vi "Serial Read Flush.vi"(11 "IO Cluster In":T1={"Error"={"status"=FALSE, "code"=0, "source"=""}, "Encoder Calibration Values"=[22, 216], "Update Calibration"=FALSE, "JPEG Resolutions"=3, "Raw Resolutions"=1, "Image Mode"=enum."RAW Gray Scale", "FPGA Ref"=refnum} {"JPEG Resolutions" items=["160x128"=3, "320x240"=5, "640x480"=7]; "Raw Resolutions" items=["80x60"=1, "160x120"=3, "128x128"=9, "128x96"=11]}) -> (3 "IO Cluster Out":T1={"Error"={"status"=FALSE, "code"=0, "source"=""}, "Encoder Calibration Values"=[22, 216], "Update Calibration"=FALSE, "JPEG Resolutions"=3, "Raw Resolutions"=1, "Image Mode"=enum."RAW Gray Scale", "FPGA Ref"=refnum} {"JPEG Resolutions" items=["160x128"=3, "320x240"=5, "640x480"=7]; "Raw Resolutions" items=["80x60"=1, "160x120"=3, "128x128"=9, "128x96"=11]})   [LabVIEW 2019]
uses:
  QNET MS IO Cluster.ctl
  <vilib>/Utility/error.llb/Error Cluster From Error Code.vi
  <vilib>/rvi/errors/niLvFpgaAdjustHostInterfaceError.vi
  <vilib>/rvi/interface/nirviMethod/nirviMethod.xnode
  <vilib>/FPGAPlugInAG/Dynamic/niLvFpga_ReadFifo_Dynamic.vi
  <vilib>/rvi/errors/niLvFpgaMergeErrorWithErrorCode.vi
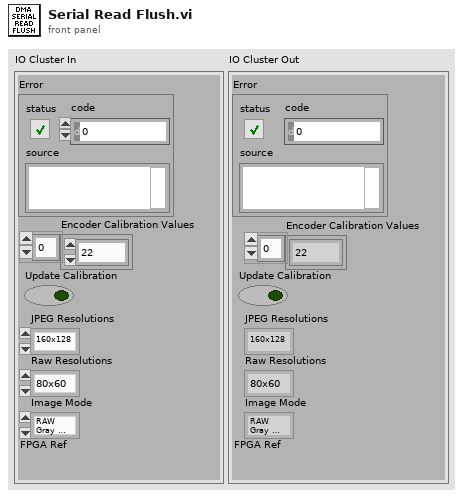
[diagram p1: front panel]
types:
  T1 = typedef "QNET MS IO Cluster.ctl" = cluster{"Error":errorcluster, "Encoder Calibration Values":i32[], "Update Calibration":bool, "JPEG Resolutions":u16, "Raw Resolutions":u16, "Image Mode":enum16{"RAW RGB", "RAW Gray Scale", "JPEG"}, "FPGA Ref":refnum<k20>}
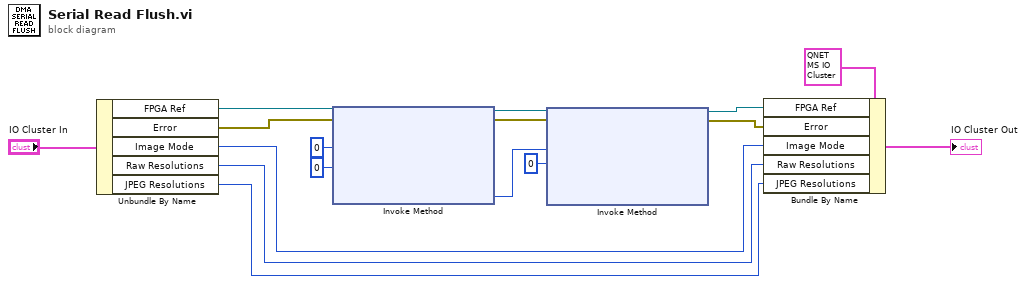
[diagram p0: block diagram]
diagram:
  n1 = Unbundle By Name("IO Cluster In") -> ("FPGA Ref"=w10:refnum<k20>, "Error"=w9:errorcluster, "Image Mode"=w6:enum16{"RAW RGB", "RAW Gray Scale", "JPEG"}, "Raw Resolutions"=w5:u16, "JPEG Resolutions"=w4:u16)
  n2 = xnode "Invoke Method"("FPGA VI引用输入"=w10, "错误输入"=w9, "Number of Elements"=u32 0, "Timeout (ms)"=0) -> ("FPGA VI引用输出"=w14:refnum<k20>, "错误输出"=w13:errorcluster, "Elements Remaining"=w12:u32)  [unwired: 1 out]
  n3 = xnode "Invoke Method"("FPGA VI引用输入"=w14, "错误输入"=w13, "Number of Elements"=w12, "Timeout (ms)"=0) -> ("FPGA VI引用输出"=w8:refnum<k20>, "错误输出"=w7:errorcluster)  [unwired: 2 out]
  n4 = Bundle By Name(cluster=T1 {"Error"={"status"=FALSE, "code"=0, "source"=""}, "Encoder Calibration Values"=[22, 216], "Update Calibration"=FALSE, "JPEG Resolutions"=3, "Raw Resolutions"=1, "Image Mode"=enum."RAW Gray Scale", "FPGA Ref"=refnum} ("IO Cluster In"), "FPGA Ref"=w8, "Error"=w7, "Image Mode"=w6, "Raw Resolutions"=w5, "JPEG Resolutions"=w4) -> (→"IO Cluster Out":T1)
